vi "Robot FPGA Utility 2.vi"() -> ()   [LabVIEW 2015]
doc: "This FPGA VI defines the functionality that is needed for the C terminal connector for the myRIO sheepdog robot project. It provides two PWM outputs, two single-line counters (for the Hall effect encoders), and digital IO needed to command the motors. It also determines a measure of the derivative of the encoder counter lines (proportional to wheel speed)."
uses:
  <vilib>/Platform/TimedLoop/XDataNode/timing_clust.ctl
  <vilib>/Platform/TimedLoop/XDataNode/nitl_modes.ctl
  <vilib>/Platform/TimedLoop/XDataNode/wakeup.ctl
  <vilib>/rvi/Emulation/niFpgaGetClockAttributes.vi
  <vilib>/rvi/Emulation/niFpgaSctlEmulationGetInTimedLoop.vi
  <vilib>/rvi/Emulation/niFpgaEmulationReportErrorSimple.vi
  <vilib>/rvi/eio/common/nirviEmuTemplateMethod_errors.vi
  <vilib>/rvi/Emulation/niFpgaCriticalErrorInLSC.vi
  <vilib>/rvi/Emulation/niFpgaProcessEmulError.vi
  <vilib>/eio/EIONode/EIONode.xnode
  <vilib>/Platform/TimedLoop/XDataNode/XDataNode.xnode
  <vilib>/eio/EIOMethodNode/EIOMethodNode.xnode
  <vilib>/Platform/TimedLoop/XDataNode/XDNodeRunTimeDep.lvlib
panel:
  in  "Stop Button":bool
  out "AccelerationX":i16
  out "Calibration counts":i16
  out "Boolean array":bool[](array[boolean])
  out "Sensor array":u8
  in  "Discharging counts":i32=20800
  in  "Motor Dir 2":bool
  in  "Motor Dir 1":bool
  out "Encoder 2 Period":u32
  out "Encoder 2 Position":i16
  out "Encoder 1 Period":u32
  out "Encoder 1 Position":i16
  in  "Reset Encoder 2":bool
  in  "Reset Encoder 1":bool
  in  "Duty Cycle Divisor":i16=30000
  in  "Duty Cycle 2":i16
  in  "Duty Cycle 1":i16
  out "SYS.RDY":bool=TRUE
  # "White 0\nBlack 1"
  # "Default : 20800"
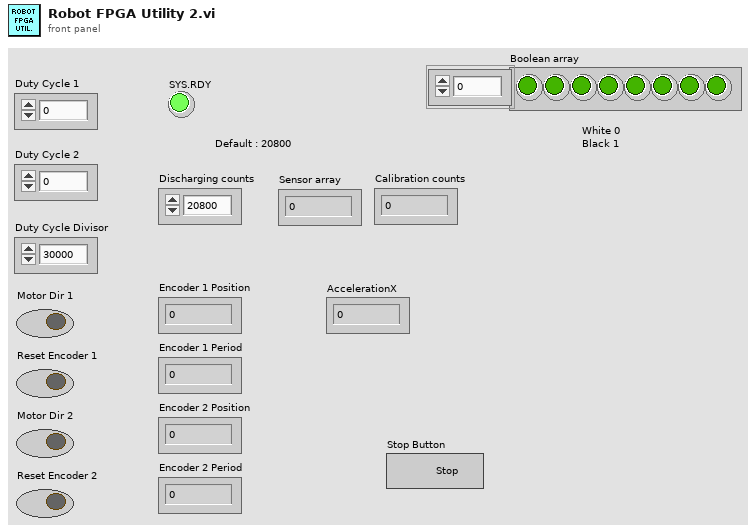
[diagram p1: front panel]
types:
  T1 = typedef "XDNodeRunTimeDep.lvlib/timing_clust.ctl" = cluster{"Expected End [f-1]":u64, "Actual End [f-1]":u64, "Finished Late? [f-1]":bool, "Expected End [i-1]":u64, "Actual End [i-1]":u64, "Finished Late? [i-1]":bool, "Expected Start [i]":u64, "Actual Start [i]":u64, "Expected Start [f]":u64, "Actual Start [f]":u64, "Source Name":string, "Structure Name":string, "Period":i64, "Deadline":i64, "Offset":i64, "Start":i64, "Priority":i32, "Timeout":i32, "Mode":T2, "Wakeup Reason":T3, "Error":errorcluster, "Source Type":string, "Secondary Source Type":string, "Global End Time":u64, "Global Start Time":u64, "Frame Duration":u64, "Iteration Duration":u64, "Assigned CPU":i32, "I/O Scan Engine Mode":u32}
  T2 = typedef "XDNodeRunTimeDep.lvlib/nitl_modes.ctl" = enum32{"No Change", "Process missed periods, maintain original phase", "Discard missed periods, maintain original phase", "Process missed periods, ignore original phase", "Discard missed periods, ignore original phase"}
  T3 = typedef "XDNodeRunTimeDep.lvlib/wakeup.ctl" = enum32{"Normal", "Aborted", "Asynchronous wakeup", "Timing source error", "Timed loop error", "Timeout"}
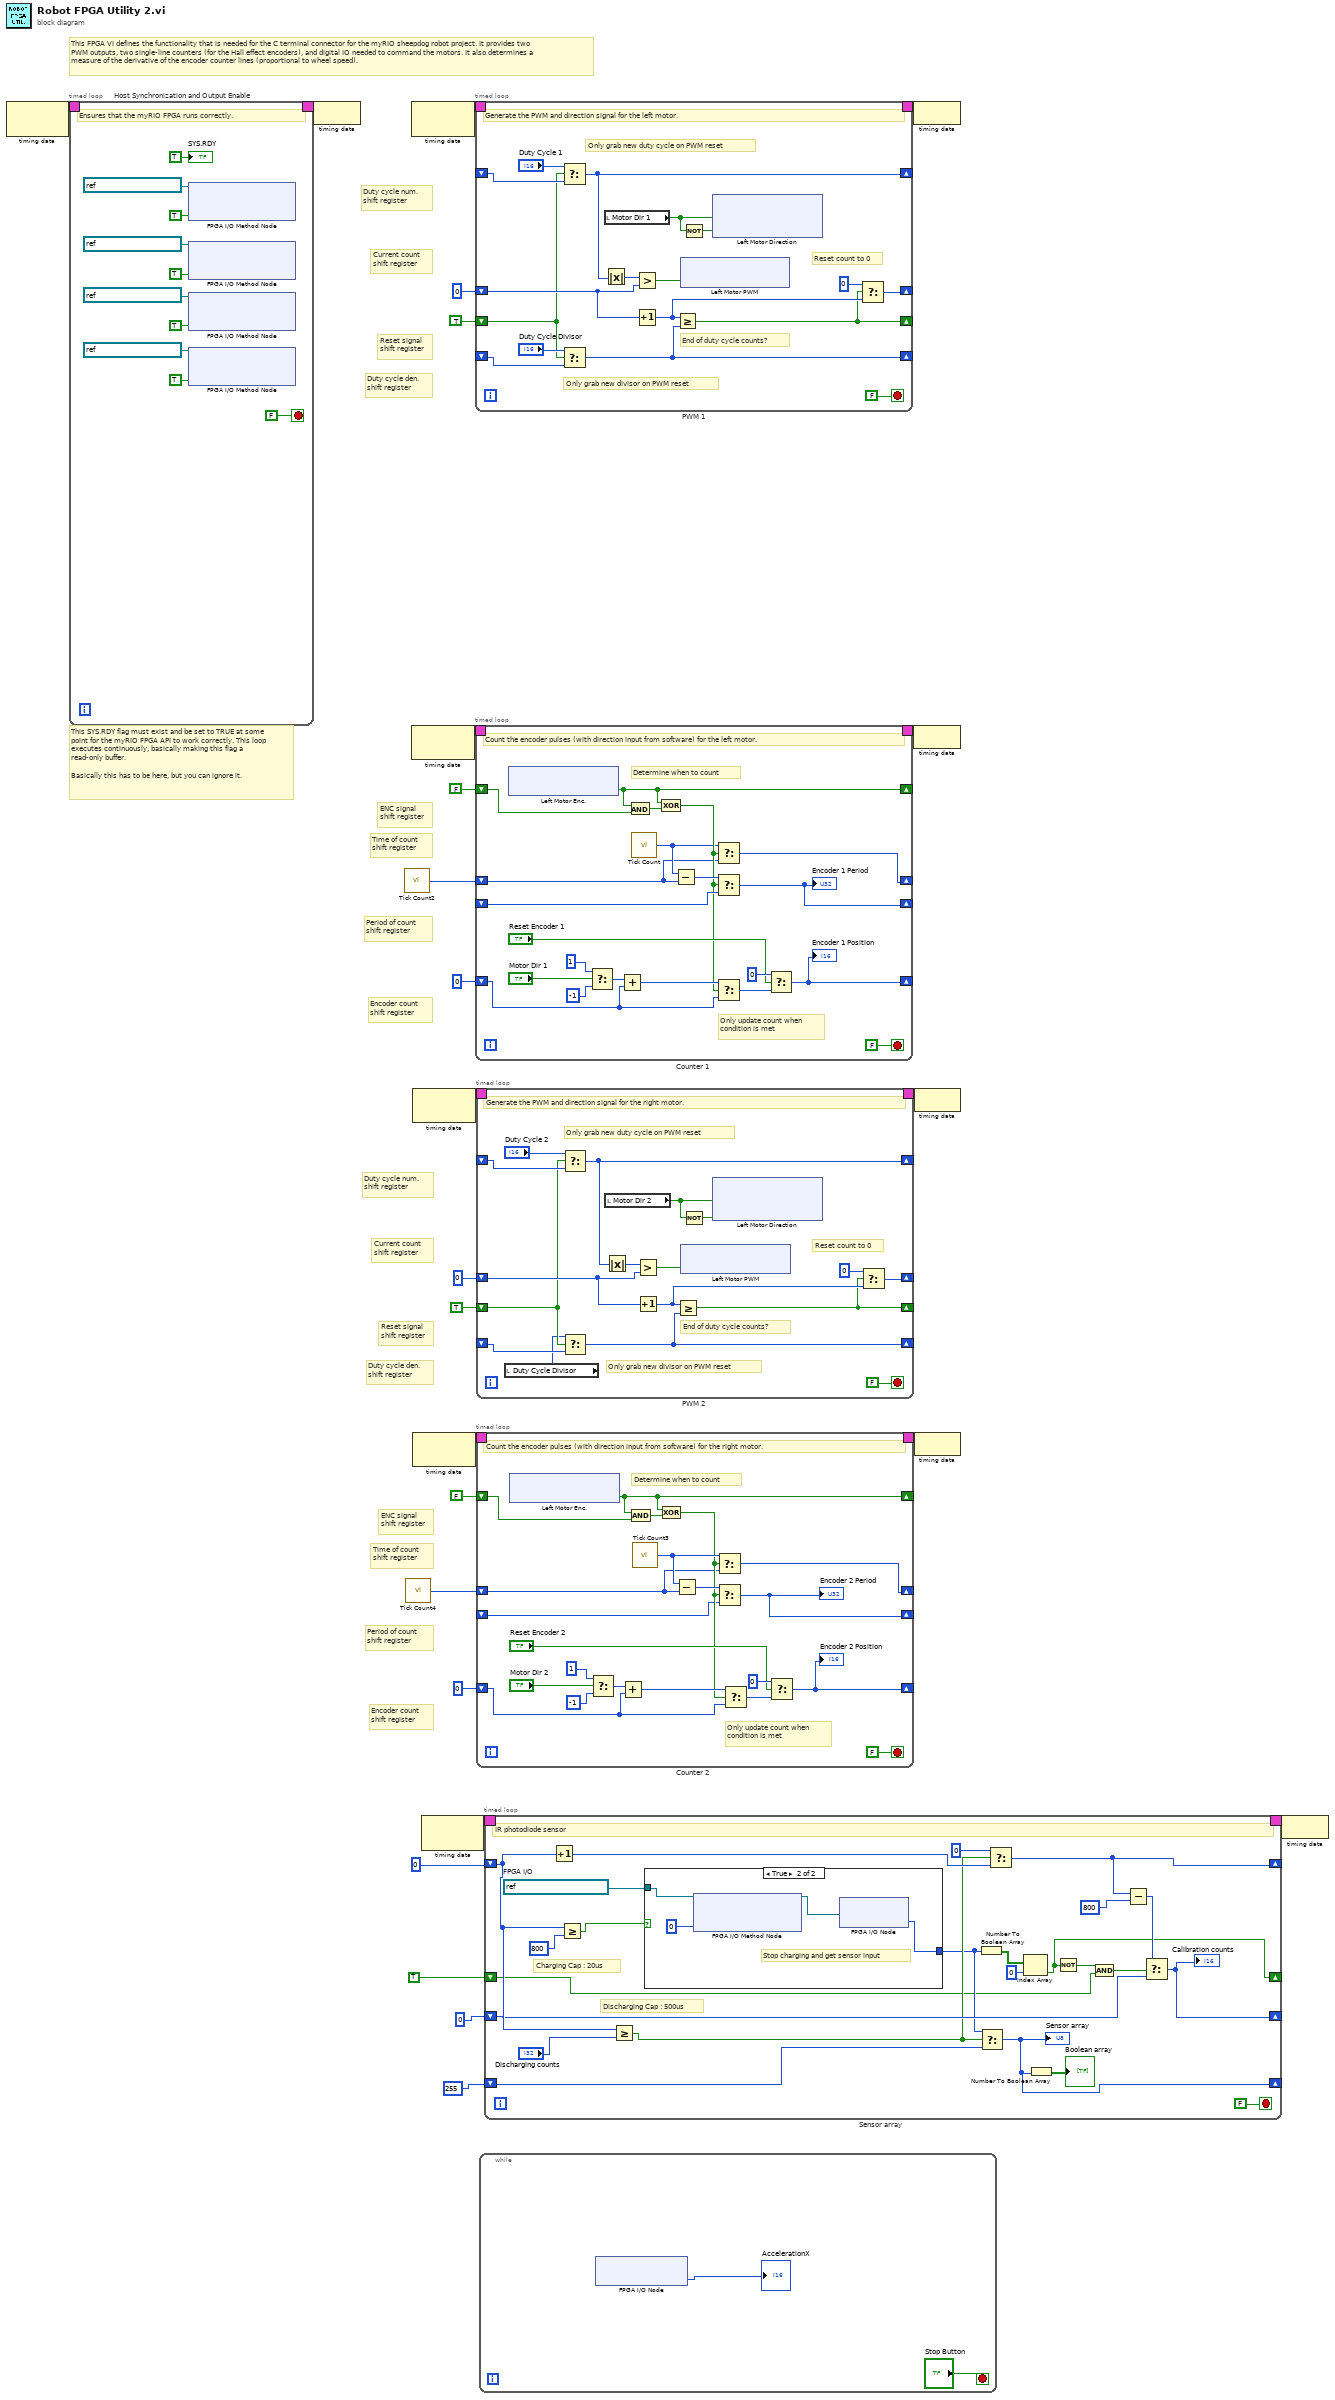
[diagram p0: block diagram]
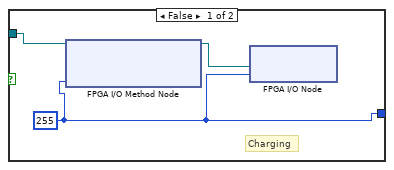
[diagram p2: hidden frame]
diagram:
  # "Period of count\nshift register"
  # "Period of count\nshift register"
  # "This SYS.RDY flag must exist and be set to TRUE at some point for the myRIO FPGA API to work correctly. This loop executes continuously, basically making this flag a read-only buffer.\n\nBasically this has to be here, but you can ignore it."
  # "Time of count\nshift register"
  # "Encoder count\nshift register"
  # "ENC signal\nshift register"
  # "Current count\nshift register"
  # "Reset signal\nshift register"
  # "Duty cycle den.\nshift register"
  # "Duty cycle num.\nshift register"
  # "Time of count\nshift register"
  # "Encoder count\nshift register"
  # "ENC signal\nshift register"
  # "Current count\nshift register"
  # "Reset signal\nshift register"
  # "Duty cycle den.\nshift register"
  # "Duty cycle num.\nshift register"
  # "This FPGA VI defines the functionality that is needed for the C terminal connector for the myRIO sheepdog robot project. It provides two PWM outputs, two single-line counters (for the Hall effect encoders), and digital IO needed to command the motors. It also determines a measure of the derivative of the encoder counter lines (proportional to wheel speed)."
  n1 = node-c288() -> (w8:T1)  [unwired: 1 in]
  n2 = timed-loop "Host Synchronization and Output Enable" {
    timing: w8 -> [_]
    timing-out: [_] -> w7
    stop <- FALSE stop-if-true
    # "Ensures that the myRIO FPGA runs correctly."
    n3 = xnode "FPGA I/O Method Node"("FPGA I/O In"=refnum<k21> "ConnectorC/DIO1", "Enable"=TRUE) -> ()  [unwired: 1 out]
    n4 = xnode "FPGA I/O Method Node"("FPGA I/O In"=refnum<k21> "ConnectorC/DIO3", "Enable"=TRUE) -> ()  [unwired: 1 out]
    n5 = xnode "FPGA I/O Method Node"("FPGA I/O In"=refnum<k21> "ConnectorC/DIO5", "Enable"=TRUE) -> ()  [unwired: 1 out]
    n6 = xnode "FPGA I/O Method Node"("FPGA I/O In"=refnum<k21> "ConnectorC/DIO7", "Enable"=TRUE) -> ()  [unwired: 1 out]
    "SYS.RDY" <- TRUE
  }
  n7 = node-c288(w7) -> ()
  n8 = call "Tick Count2"() -> ("Tick Count(Ticks)"=w20:u32)
  n9 = call "Tick Count4"() -> ("Tick Count(Ticks)"=w11:u32)
  n10 = node-c288() -> (w26:T1)  [unwired: 1 in]
  n11 = node-c288() -> (w22:T1)  [unwired: 1 in]
  n12 = node-c288() -> (w17:T1)  [unwired: 1 in]
  n13 = node-c288() -> (w15:T1)  [unwired: 1 in]
  n14 = node-c288() -> (w6:T1)  [unwired: 1 in]
  n15 = timed-loop "PWM 1" {
    timing: w26 -> [_]
    timing-out: [_] -> w25
    shift-right: [w53] -> _
    shift-left: _ -> [w54]
    shift-right: [w47] -> _
    shift-left: i16 0 -> [w50]
    shift-right: [w45] -> _
    shift-left: TRUE -> [w43]
    shift-right: [w42] -> _
    shift-left: _ -> [w41]
    stop <- FALSE stop-if-true
    # "Only grab new divisor on PWM reset"
    # "End of duty cycle counts?"
    # "Reset count to 0"
    # "Only grab new duty cycle on PWM reset"
    # "Generate the PWM and direction signal for the left motor."
    n16 = Select(t="Duty Cycle 1", s=w43, f=w54) -> (s? t:f=w53:i16)
    n17 = Select(t="Duty Cycle Divisor", s=w43, f=w41) -> (s? t:f=w42:i16)
    n18 = local read "Motor Dir 1"() -> (w39:bool)
    n19 = Absolute Value(x=w53) -> (abs(x)=w52:i16)
    n20 = Greater?(x=w52, y=w50) -> (0:w51:bool)
    n21 = Increment(x=w50) -> (x+1=w49:i16)
    n22 = Greater Or Equal?(x=w49, y=w42) -> (x >= y?=w45:bool)
    n23 = xnode "Left Motor PWM"("ConnectorC/DIO3"=w51) -> ()  [unwired: 1 in, 1 out]
    n24 = Not(x=w39) -> (.not. x?=w40:bool)
    n25 = xnode "Left Motor Direction"("ConnectorC/DIO0"=w39, "ConnectorC/DIO1"=w40) -> ()  [unwired: 2 in, 2 out]
    n26 = Select(t=i16 0, s=w45, f=w49) -> (s? t:f=w47:i16)
  }
  n27 = timed-loop "Counter 1" {
    timing: w22 -> [_]
    timing-out: [_] -> w21
    shift-right: [w69] -> _
    shift-left: i16 0 ("t") -> [w70]
    shift-right: [w66] -> _
    shift-left: FALSE ("ConnectorC/DIO2") -> [w68]
    shift-right: [w58] -> _
    shift-left: w20 -> [w59]
    shift-right: [w62] -> _
    shift-left: _ -> [w63]
    stop <- FALSE stop-if-true
    # "Determine when to count"
    # "Only update count when\ncondition is met"
    # "Count the encoder pulses (with direction input from software) for the left motor."
    n28 = xnode "Left Motor Enc."() -> ("ConnectorC/DIO2"=w66:bool)  [unwired: 1 in, 1 out]
    n29 = Select(t=i16 1, s="Motor Dir 1", f=i16 -1) -> (s? t:f=w75:i16)
    n30 = Add(x=w75, y=w70) -> (x+y=w74:i16)
    n31 = And(x=w66, y=w68) -> (x .and. y?=w67:bool)
    n32 = call "Tick Count"() -> ("Tick Count(Ticks)"=w60:u32)
    n33 = Exclusive Or(1:w67, 2:w66) -> (0:w61:bool)
    n34 = Subtract(x=w60, y=w59) -> (x-y=w65:u32)
    n35 = Select(t=w60, s=w61, f=w59) -> (s? t:f=w58:u32)
    n36 = Select(t=w65, s=w61, f=w63) -> (s? t:f=w62:u32)
    "Encoder 1 Period" <- w62
    n37 = Select(t=w74, s=w61, f=w70) -> (s? t:f=w73:i16)
    n38 = Select(t=i16 0, s="Reset Encoder 1", f=w73) -> (s? t:f=w69:i16)
    "Encoder 1 Position" <- w69
  }
  n39 = timed-loop "PWM 2" {
    timing: w17 -> [_]
    timing-out: [_] -> w16
    shift-right: [w96] -> _
    shift-left: _ -> [w97]
    shift-right: [w90] -> _
    shift-left: i16 0 -> [w93]
    shift-right: [w88] -> _
    shift-left: TRUE -> [w87]
    shift-right: [w86] -> _
    shift-left: _ -> [w85]
    stop <- FALSE stop-if-true
    # "Only grab new divisor on PWM reset"
    # "End of duty cycle counts?"
    # "Reset count to 0"
    # "Only grab new duty cycle on PWM reset"
    # "Generate the PWM and direction signal for the right motor."
    n40 = local read "Duty Cycle Divisor"() -> (w83:i16)
    n41 = Select(t="Duty Cycle 2", s=w87, f=w97) -> (s? t:f=w96:i16)
    n42 = Select(t=w83, s=w87, f=w85) -> (s? t:f=w86:i16)
    n43 = local read "Motor Dir 2"() -> (w82:bool)
    n44 = Absolute Value(x=w96) -> (abs(x)=w95:i16)
    n45 = Greater?(x=w95, y=w93) -> (0:w94:bool)
    n46 = Increment(x=w93) -> (x+1=w92:i16)
    n47 = Greater Or Equal?(x=w92, y=w86) -> (x >= y?=w88:bool)
    n48 = xnode "Left Motor PWM"("ConnectorC/DIO7"=w94) -> ()  [unwired: 1 in, 1 out]
    n49 = Not(x=w82) -> (.not. x?=w81:bool)
    n50 = xnode "Left Motor Direction"("ConnectorC/DIO4"=w82, "ConnectorC/DIO5"=w81) -> ()  [unwired: 2 in, 2 out]
    n51 = Select(t=i16 0, s=w88, f=w92) -> (s? t:f=w90:i16)
  }
  n52 = timed-loop "Counter 2" {
    timing: w15 -> [_]
    timing-out: [_] -> w14
    shift-right: [w109] -> _
    shift-left: i16 0 ("t") -> [w114]
    shift-right: [w111] -> _
    shift-left: FALSE ("ConnectorC/DIO2") -> [w113]
    shift-right: [w100] -> _
    shift-left: w11 -> [w103]
    shift-right: [w102] -> _
    shift-left: _ -> [w101]
    stop <- FALSE stop-if-true
    # "Determine when to count"
    # "Only update count when\ncondition is met"
    # "Count the encoder pulses (with direction input from software) for the right motor."
    n53 = xnode "Left Motor Enc."() -> ("ConnectorC/DIO6"=w111:bool)  [unwired: 1 in, 1 out]
    n54 = Select(t=i16 1, s="Motor Dir 2", f=i16 -1) -> (s? t:f=w118:i16)
    n55 = Add(x=w118, y=w114) -> (x+y=w117:i16)
    n56 = And(x=w111, y=w113) -> (x .and. y?=w112:bool)
    n57 = call "Tick Count3"() -> ("Tick Count(Ticks)"=w105:u32)
    n58 = Exclusive Or(1:w112, 2:w111) -> (0:w104:bool)
    n59 = Subtract(x=w105, y=w103) -> (x-y=w106:u32)
    n60 = Select(t=w105, s=w104, f=w103) -> (s? t:f=w100:u32)
    n61 = Select(t=w106, s=w104, f=w101) -> (s? t:f=w102:u32)
    "Encoder 2 Period" <- w102
    n62 = Select(t=w117, s=w104, f=w114) -> (s? t:f=w116:i16)
    n63 = Select(t=i16 0, s="Reset Encoder 2", f=w116) -> (s? t:f=w109:i16)
    "Encoder 2 Position" <- w109
  }
  n64 = while {
    stop <- "Stop Button" stop-if-true
    n65 = xnode "FPGA I/O Node"() -> ("AccelerationX"=→"AccelerationX":i16)  [unwired: 1 in, 1 out]
  }
  n66 = timed-loop "Sensor array" {
    timing: w6 -> [_]
    timing-out: [_] -> w5
    shift-right: [w131] -> _
    shift-left: i16 0 -> [w144]
    shift-right: [w140] -> _
    shift-left: i16 255 ("Enable") -> [w128]
    shift-right: [w130] -> _
    shift-left: i16 0 ("Enable") -> [w134]
    shift-right: [w129] -> _
    shift-left: TRUE -> [w126]
    stop <- FALSE stop-if-true
    w148 = refnum<k21> "ConnectorA/DIO7:0"  # FPGA I/O
    # "Discharging Cap : 500us"
    # "Charging Cap : 20us"
    # "IR photodiode sensor"
    n67 = Increment(x=w144) -> (x+1=w142:i16)
    n68 = Greater Or Equal?(x=w144, y=i16 800) -> (x >= y?=w146:bool)
    n69 = Greater Or Equal?(x=w144, y="Discharging counts") -> (x >= y?=w132:bool)
    n70 = case shown="True" w146 {
      tunnel: w148 -> [w151 w155]
      tunnel: [w149 w153] -> w127
      frame False {
        w149 = i16 255
        # "Charging"
        n71 = xnode "FPGA I/O Method Node"("FPGA I/O In"=w151, "Enable"=w149) -> ("FPGA I/O Out"=w150:refnum<k21>)
        n72 = xnode "FPGA I/O Node"("I/O Item"=w149, "FPGA I/O In"=w150) -> ()  [unwired: 1 out]
      }
      frame True {
        # "Stop charging and get sensor input"
        n73 = xnode "FPGA I/O Method Node"("FPGA I/O In"=w155, "Enable"=u8 0) -> ("FPGA I/O Out"=w154:refnum<k21>)
        n74 = xnode "FPGA I/O Node"("FPGA I/O In"=w154) -> ("I/O Item"=w153:u8)  [unwired: 1 out]
      }
    }
    n75 = Number To Boolean Array(number=w127) -> (Boolean array=w139:bool[])
    n76 = Select(t=w127, s=w132, f=w128) -> (s? t:f=w140:i16)
    "Sensor array" <- w140
    n77 = Select(t=u8 0 ("Enable"), s=w132, f=w142) -> (s? t:f=w131:i16)
    n78 = Index Array(array=w139, index=0) -> (element=w129:bool)
    n79 = Number To Boolean Array(number=w140) -> (Boolean array=→"Boolean array":bool[])
    n80 = Not(x=w129) -> (.not. x?=w133:bool)
    n81 = And(x=w133, y=w126) -> (x .and. y?=w135:bool)
    n82 = Subtract(x=w131, y=800 ("index")) -> (x-y=w136:i32)
    n83 = Select(t=w136, s=w135, f=w134) -> (s? t:f=w130:i32)
    "Calibration counts" <- w130
  }
  n84 = node-c288(w25) -> ()
  n85 = node-c288(w21) -> ()
  n86 = node-c288(w16) -> ()
  n87 = node-c288(w14) -> ()
  n88 = node-c288(w5) -> ()
